vi "GetDeviceInformation.vi"(3 "error in (no error)":errorcluster, 4 "device module":string, 5 "physical channels":string="DemoDevice,BID#0/ai0", 6 "task in":i32) -> (0 "错误输出":errorcluster, 1 "输出簇":T1, 2 "task out":i32)   [LabVIEW 2012]
uses:
  <userlib>/DAQNavi Polymorphic VI/configure/DAQNavi Get Property/AI/DAQNaviGet_AI_ChannelStart.vi
  <userlib>/DAQNavi Polymorphic VI/configure/DAQNavi Get Property/AI/DAQNaviGet_AI_ValueRange_Information.vi
  <userlib>/DAQNavi Polymorphic VI/configure/DAQNavi Get Property/AI/DAQNaviGet_AI_ConvertClock_Rate.vi
  <userlib>/DAQNavi Polymorphic VI/configure/DAQNavi Get Property/AI/DAQNaviGet_AI_ChannelCount.vi
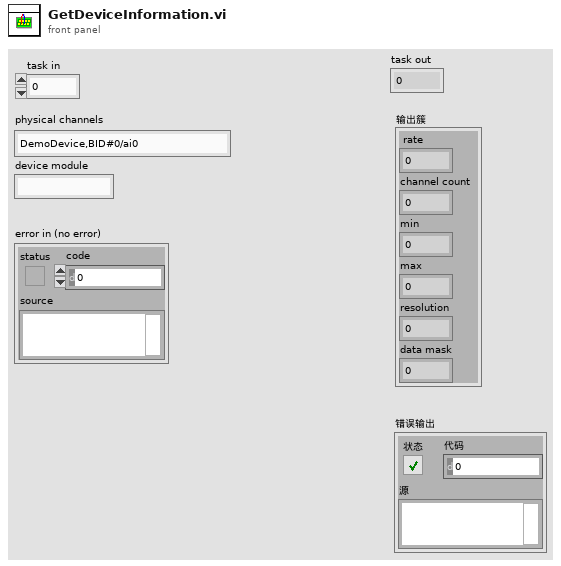
[diagram p1: front panel]
types:
  T1 = cluster{" rate":dbl, "channel count":i32, "min":dbl, "max":dbl, "resolution":i32, "data mask":i32}
  T2 = cluster{" rate":dbl, "channel count":i32, "min":dbl, "max":dbl, "int value":i32, "int value":i32}
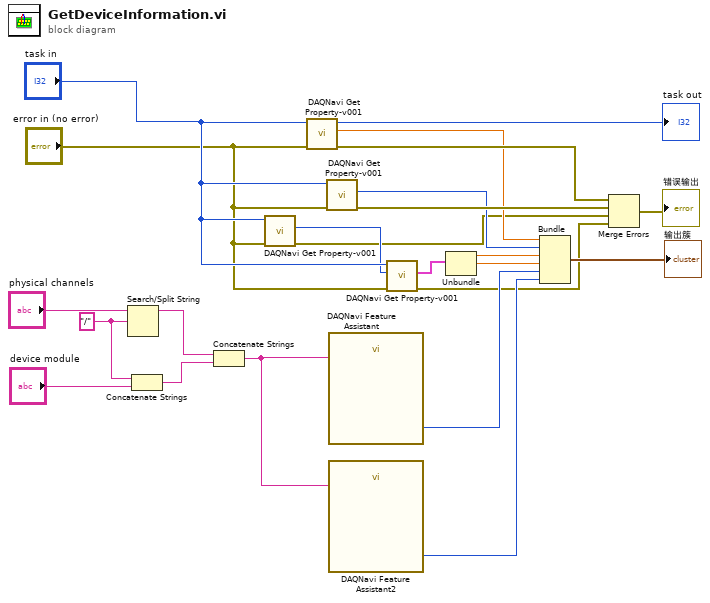
[diagram p0: block diagram]
diagram:
  w21 = "/" ("搜索字符串")
  n1 = Search/Split String(string="physical channels", search string/char (-)=w21) -> (substring before match=w23:string)  [unwired: 1 in, 2 out]
  n2 = Concatenate Strings(w21, "device module") -> (w20:string)
  n3 = Concatenate Strings(w23, w20) -> (w22:string)
  n4 = call-poly <userlib>:"DAQNavi Get Property-v001.vi"("error in (no error)"="error in (no error)", "task in"="task in") -> ("error out"=w2:errorcluster, "start channel"=w4:i32)  [unwired: 7 in, 1 out]
  n5 = call-poly <userlib>:"DAQNavi Get Property-v001.vi"("error in (no error)"="error in (no error)", "task in"="task in") -> ("error out"=w17:errorcluster, "rate"=w13:dbl, "task out"=→"task out":i32)  [unwired: 7 out]
  n6 = call-poly <userlib>:"DAQNavi Get Property-v001.vi"("error in (no error)"="error in (no error)", "task in"="task in") -> ("error out"=w18:errorcluster, "channel count"=w3:i32)  [unwired: 7 in, 1 out]
  n7 = call "DAQNavi Feature Assistant"("device"=w22) -> ("int value"=w12:i32)  [unwired: 14 in]
  n8 = call "DAQNavi Feature Assistant2"("device"=w22) -> ("int value"=w11:i32)  [unwired: 14 in]
  n9 = call-poly <userlib>:"DAQNavi Get Property-v001.vi"("error in (no error)"="error in (no error)", "channel"=w4, "task in"="task in") -> ("error out"=w1:errorcluster, "Information"=w10:cluster{"min":dbl, "max":dbl, "unit":string})  [unwired: 6 in, 1 out]
  n10 = Unbundle(w10) -> ("min"=w9:dbl, "max"=w8:dbl)  [unwired: 1 out]
  n11 = Bundle("rate"=w13, "channel count"=w3, "min"=w9, "max"=w8, "int value"=w12, "int value"=w11) -> (→"输出簇":T2)  [unwired: 1 in]
  n12 = Merge Errors(w17, w18, w2, w1) -> (→"错误输出":errorcluster)
